vi "New.vi"(8 "error in (no error)":errorcluster, 11 "reference in":refnum<class "Dynamic TestSuite.lvclass">) -> (0 "error out":errorcluster, 3 "reference out":refnum<class "Dynamic TestSuite.lvclass">)   [LabVIEW 2011, in "Dynamic TestSuite.lvclass"]
uses:
  Dynamic TestSuite.lvclass
  Classes/TestCase/TestCase.lvclass
  WaitOnTestComplete/WaitOnTestComplete.lvclass
  DoNotWaitOnTestComplete/DoNotWaitOnTestComplete.lvclass
  LocationOutsideClassRoot/LocationOutsideClassRoot.lvclass
  Classes/TestSuite/TestSuite.lvclass
  Classes/TestLoader/TestLoader.lvclass
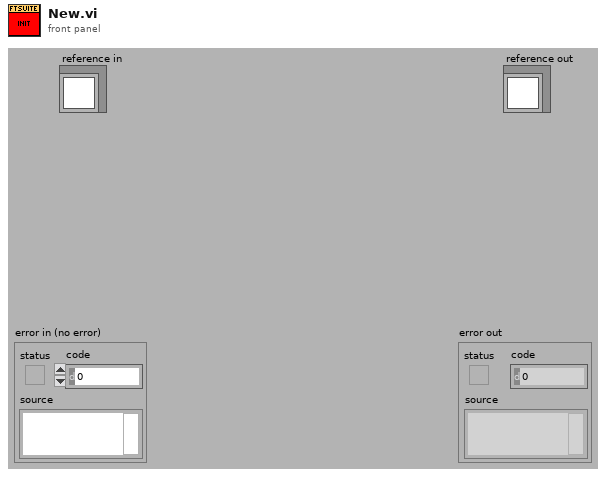
[diagram p1: front panel]
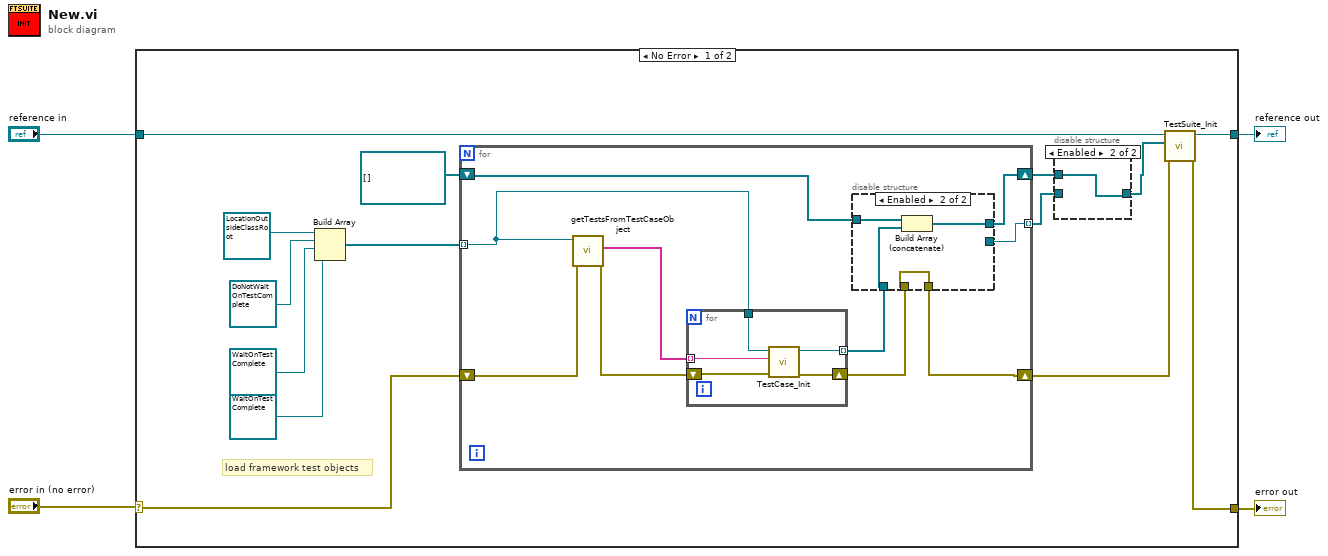
[diagram p0: block diagram]
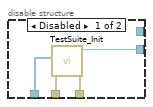
[diagram p3: hidden frame]
diagram:
  n1 = case shown="No Error" "error in (no error)" {
    selector: "error in (no error)" -> [w15 w44]
    tunnel: [w14 w45] -> w4
    tunnel: "reference in" -> [w9 w45]
    tunnel: [w18 w44] -> w1
    frame No Error {
      # "load framework test objects"
      n2 = Build Array(refnum<class "LocationOutsideClassRoot.lvclass"> refnum ("LocationOutsideClassRoot.lvclass"), refnum<class "DoNotWaitOnTestComplete.lvclass"> refnum ("DoNotWaitOnTestComplete.lvclass"), refnum<class "WaitOnTestComplete.lvclass"> refnum ("WaitOnTestComplete.lvclass"), refnum<class "WaitOnTestComplete.lvclass"> refnum ("WaitOnTestComplete.lvclass")) -> (w16:refnum<class "TestCase.lvclass">[])
      n3 = for {
        shift-right: [w24] -> w13
        shift-left: w15 -> [w29]
        tunnel: w16 -> [w30] mode=indexing
        tunnel: [w21] -> w6 mode=indexing
        shift-right: [w22] -> w5
        shift-left: refnum<class "TestCase.lvclass">[] [] -> [w23]
        n4 = call "getTestsFromTestCaseObject.vi"("error in"=w29, "Test in"=w30) -> ("error out"=w27:errorcluster, "Test Method Names"=w28:string[])  [unwired: 7 in, 1 out]
        n5 = for {
          tunnel: w30 -> [w39]
          tunnel: w28 -> [w43] mode=indexing
          shift-right: [w41] -> w25
          shift-left: w27 -> [w42]
          tunnel: [w40] -> w26 mode=indexing
          n6 = call "TestCase_Init.vi"("error in (no error)"=w42, "methodName (\"runTest\")"=w43, "TestCase in"=w39) -> ("error out"=w41:errorcluster, "TestCase out"=w40:refnum<class "TestCase.lvclass">)  [unwired: 7 in]
        }
        n7 = disable-structure shown="Enabled" {
          disable-tunnel: w26 -> [w34 w37]
          disable-tunnel: w25 -> [w33 w35]
          disable-tunnel: [w32 w35] -> w24
          disable-tunnel: [_ w36] -> w22
          disable-tunnel: w23 -> [_ w38]
          disable-tunnel: [w31 _] -> w21
          frame Disabled {
            n8 = call "TestSuite_Init.vi"("error in (no error)"=w33, "tests (none)"=w34) -> ("error out"=w32:errorcluster, "TestSuite out"=w31:refnum<class "TestSuite.lvclass">)  [unwired: 8 in]
          }
          frame Enabled {
            n9 = Build Array (concatenate)(w38, w37) -> (w36:refnum<class "TestCase.lvclass">[])
          }
        }
      }
      n10 = disable-structure shown="Enabled" {
        disable-tunnel: [w19 w20] -> w7
        disable-tunnel: w6 -> [w19 _]
        disable-tunnel: w5 -> [_ w20]
        frame Disabled {
        }
        frame Enabled {
        }
      }
      n11 = call "TestSuite_Init.vi"("error in (no error)"=w13, "tests (none)"=w7, "TestSuite in"=w9) -> ("error out"=w18:errorcluster, "TestSuite out"=w14:refnum<class "Dynamic TestSuite.lvclass">)  [unwired: 7 in]
    }
    frame Error {
    }
  }
  "reference out" <- w4
  "error out" <- w1
